vi "PID_regulator.vi"(0 "Integral in":dbl, 4 "Punkt rownowagi":dbl, 8 "Ki":dbl, 9 "Kd":dbl, 10 "Kp":dbl, 11 "IN":dbl[](array[numeric])) -> (1 "Integral out":dbl, 3 "OUT":dbl)   [LabVIEW 2019]
uses:
  <vilib>/Analysis/baseanly.llb/Mean (DBL).vi
  <vilib>/Analysis/NI_AALBase.lvlib
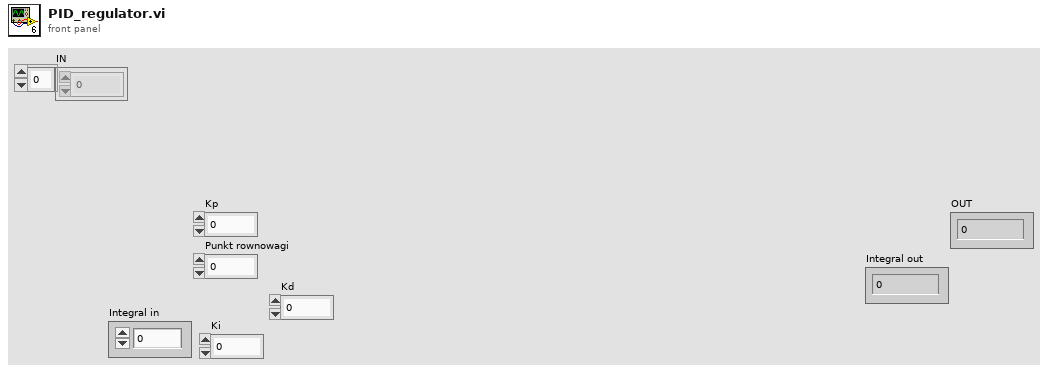
[diagram p1: front panel]
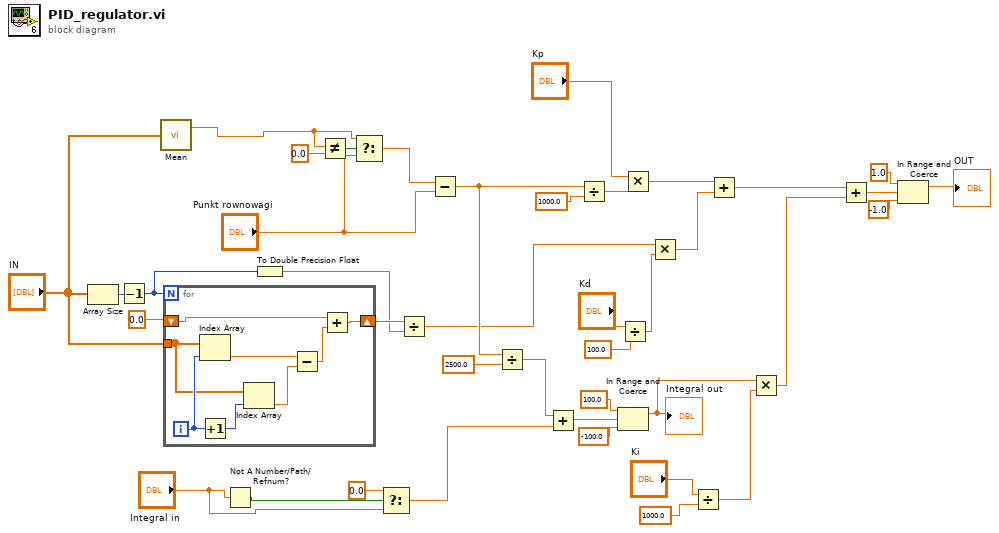
[diagram p0: block diagram]
diagram:
  n1 = Array Size(array="IN") -> (size(s)=w9:i32)
  n2 = Decrement(x=w9) -> (x-1=w6:i32)
  n3 = call-poly <vilib>:"Mean.vi"("X"="IN") -> ("mean"=w2:dbl)  [unwired: 1 out]
  n4 = for {
    N: w6 -> [_]
    tunnel: "IN" -> [w46]
    shift-right: [w41] -> w7
    shift-left: 0.0 ("x") -> [w43]
    i -> [w48]
    n5 = Index Array(array=w46, index=w48) -> (element=w45:dbl)
    n6 = Increment(x=w48) -> (x+1=w47:i32)
    n7 = Index Array(array=w46, index=w47) -> (element=w44:dbl)
    n8 = Subtract(x=w45, y=w44) -> (x-y=w42:dbl)
    n9 = Add(x=w43, y=w42) -> (x+y=w41:dbl)
  }
  n10 = Not A Number/Path/Refnum?(number/path/refnum="Integral in") -> (NaN/Path/Refnum?=w18:bool)
  n11 = To Double Precision Float(number=w6) -> (double precision float=w5:dbl)
  n12 = Not Equal?(x=w2, y=0.0) -> (x != y?=w22:bool)
  n13 = Select(t=w2, s=w22, f="Punkt rownowagi") -> (s? t:f=w23:dbl)
  n14 = Select(t=0.0, s=w18, f="Integral in") -> (s? t:f=w19:dbl)
  n15 = Divide(x=w7, y=w5) -> (x/y=w4:dbl)
  n16 = Subtract(x=w23, y="Punkt rownowagi") -> (x-y=w28:dbl)
  n17 = Divide(x=w28, y=2500.0) -> (x/y=w30:dbl)
  n18 = Add(x=w30, y=w19) -> (x+y=w25:dbl)
  n19 = Divide(x=w28, y=1000.0) -> (x/y=w27:dbl)
  n20 = In Range and Coerce(upper limit=100.0, x=w25, lower limit=-100.0) -> (coerced(x)=w1:dbl)  [unwired: 1 out]
  "Integral out" <- w1
  n21 = Divide(x="Kd", y=100.0) -> (x/y=w13:dbl)
  n22 = Multiply(x="Kp", y=w27) -> (x*y=w39:dbl)
  n23 = Multiply(x=w4, y=w13) -> (x*y=w38:dbl)
  n24 = Divide(x="Ki", y=1000.0) -> (x/y=w10:dbl)
  n25 = Add(x=w39, y=w38) -> (x+y=w37:dbl)
  n26 = Multiply(x=w1, y=w10) -> (x*y=w24:dbl)
  n27 = Add(x=w37, y=w24) -> (x+y=w34:dbl)
  n28 = In Range and Coerce(upper limit=1.0, x=w34, lower limit=-1.0) -> (coerced(x)=→"OUT":dbl)  [unwired: 1 out]
